vi "Control Spring.vi"   [LabVIEW 2020]
uses:
  Framework/Robot Global Data.vi
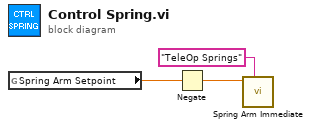
[diagram p0: block diagram]
diagram:
  n1 = global read "Robot Global Data.vi" "Spring Arm Setpoint"() -> (w2:dbl)
  n2 = Negate(x=w2) -> (-x=w3:dbl)
  n3 = call "Spring Arm Immediate.vi"("Description"="TeleOp Springs", "Setpoint"=w3) -> ()  [unwired: 9 in, 1 out]
